vi "rqcBob QKey Processing.vi"(0 "rqcBob ServiceNET in":T1, 5 "Correct indices":u32[](array[numeric]), 7 "Raw Bob's data":u8[](array[numeric]), 9 "data valid":bool, 11 "error in":errorcluster) -> (4 "rqcBob ServiceNET out":T1, 6 "Incorrect Alice's data":bool, 8 "Bob's Key:":string="010100110101111110011011110000111111100101101001011100110010001011010011011001010000111101100001111011001111110010010110111100010001111011001000011001001101011000010111001010101110111010010000110011001101101100100101111100001111001011011110000010010101011001111010111001111100111110100100111011110001110101001100010011010001011011101010101000100011010101011010010001111110100010011010011001101101101000001100010110011001101001010101011000110010101100111101110101110011110100101100100001100100001101100001110010011000001101111001111110101101001010000110011100000011111101100010010100111000101011100110111010011100100000110000100110111101100000011011010011110000111011110111001101110001101011100111000010001001011000101100001110011001000100110101110010100000011011000001100111000101000100001110001001001011101100101101111000011101000111001110111000000101101000101011110101001101000001001000010011001010000011111111010010010001111011111001110001010100000010001000000101000000100101011010110100010111110111011110001100101010110010011101001010001100100000110000001111110101000001010000110001000011101110100110001000001100010101001000", 15 "error out":errorcluster)   [LabVIEW 2018]
uses:
  Shared/Shared Host Lib/rqc ServiceNET/Bob/Custom Controls/rqcBob ServiceNET control.ctl
  Shared/Shared Host Lib/rqc ServiceNET/Custom Controls/rqc ServiceNET command.ctl
  Shared/Shared Host Lib/rqc ServiceNET/Bob/rqcBob Send Data/rqcBob ServiceNET Send Data U8.vi
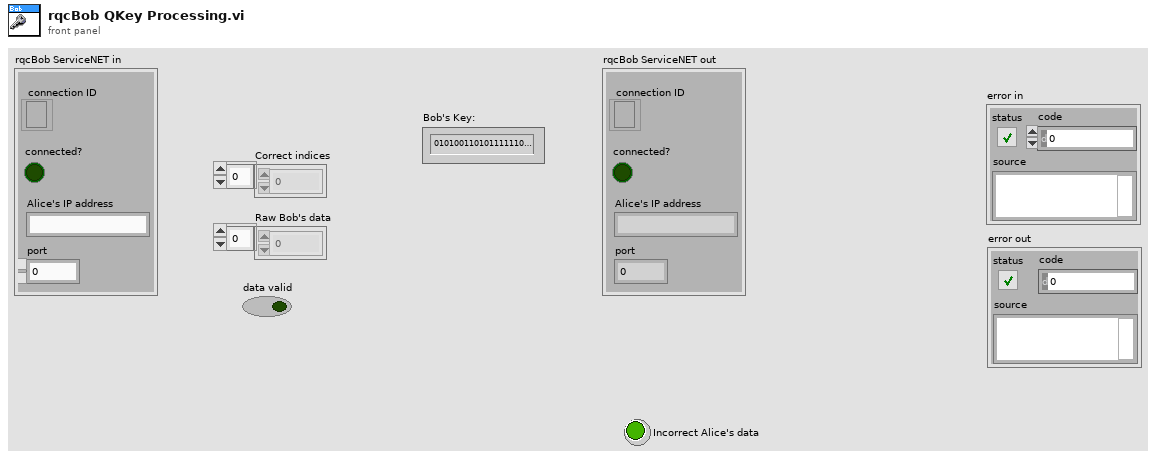
[diagram p1: front panel]
types:
  T1 = typedef "rqcBob ServiceNET control.ctl" = cluster{"connection ID":refnum<k5>, "connected?":bool, "Alice's IP address":string, "port":u16}
  T2 = typedef "rqc ServiceNET command.ctl" = enum8{"NONE", "READY", "START", "PING", "SEND KEY", "WRITE KEY", "WRITE AND SAVE KEY"}
  T3 = enum16{"open", "replace", "create", "open or create", "replace or create", "replace or create with confirmation"}
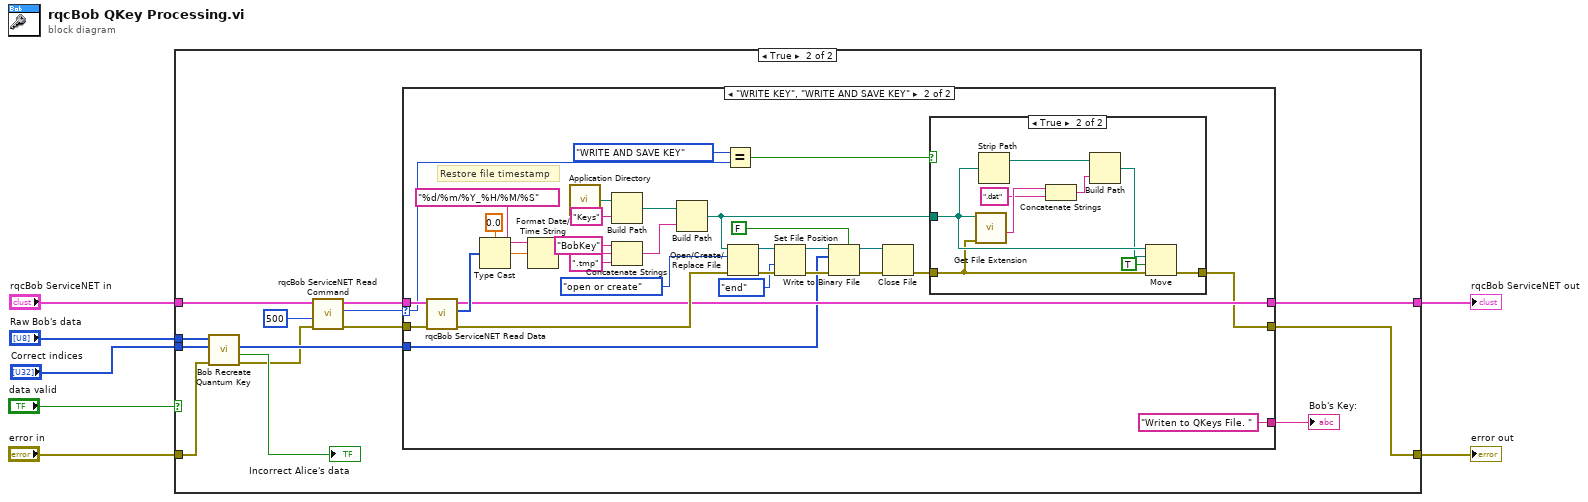
[diagram p0: block diagram]
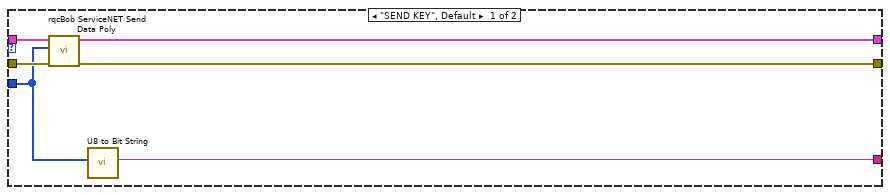
[diagram p3: hidden frame]
diagram:
  n1 = case shown="True" "data valid" {
    tunnel: "Raw Bob's data" -> [_ w23]
    tunnel: "Correct indices" -> [_ w22]
    tunnel: "error in" -> [w9 w21]
    tunnel: [w9 w18] -> w2
    tunnel: "rqcBob ServiceNET in" -> [w8 w16]
    tunnel: [w8 w19] -> w6
    frame False {
    }
    frame True {
      n2 = call "Bob Recreate Quantum Key.vi"("error in"=w21, "Correct Measurements Indexes in"=w22, "Raw Data in"=w23) -> ("error out"=w15:errorcluster, "Incorrect Alice's data"=→"Incorrect Alice's data":bool, "Sifted Key out"=w17:u8[])  [unwired: 6 in]
      n3 = call "rqcBob ServiceNET Read Command.vi"("error in"=w15, "timeout ms (50)"=500, "rqcBob ServiceNET in"=w16) -> ("error out"=w12:errorcluster, "command"=w14:T2, "rqcBob ServiceNET out"=w13:T1)  [unwired: 5 in, 1 out]
      n4 = case shown="\"WRITE KEY\", \"WRITE AND SAVE KEY\"" w14 {
        selector: w14 -> [_ w34]
        tunnel: [w29 w36] -> w19
        tunnel: [w28 w35] -> w18
        tunnel: w17 -> [w25 w31]
        tunnel: w13 -> [w27 w61]
        tunnel: w12 -> [w26 w60]
        tunnel: [w24 "Writen to QKeys File. " ("String out")] -> w11
        frame "SEND KEY", Default {
          n5 = call-poly "rqcBob ServiceNET Send Data Poly.vi"("error in"=w26, "Data"=w25, "rqcBob ServiceNET in"=w27) -> ("error out"=w28:errorcluster, "rqcBob ServiceNET out"=w29:T1)  [unwired: 7 in]
          n6 = call "U8 to Bit String.vi"("U8 in"=w25) -> ("String out"=w24:string)  [unwired: 10 in]
        }
        frame "WRITE KEY", "WRITE AND SAVE KEY" {
          # "Restore file timestamp"
          n7 = call "rqcBob ServiceNET Read Data.vi"("error in"=w60, "rqcBob ServiceNET in"=w61) -> ("error out"=w37:errorcluster, "Data"=w59:u32[], "rqcBob ServiceNET out"=w36:T1)  [unwired: 6 in, 1 out]
          n8 = Type Cast(type=0.0, x=w59) -> (*(type *) &x=w56:dbl)
          n9 = Format Date/Time String(time format string (%c)="%d/%m/%Y_%H/%M/%S", seconds (now)=w56) -> (date/time string=w55:string)  [unwired: 1 in]
          n10 = call <vilib>:"Application Directory.vi"() -> ("Application Directory"=w52:path)
          n11 = Build Path(base path=w52, name or relative path="Keys") -> (appended path=w49:path)
          n12 = Concatenate Strings("BobKey" ("string"), w55, ".tmp" ("string")) -> (w50:string)
          n13 = Build Path(base path=w49, name or relative path=w50) -> (appended path=w38:path)
          n14 = Equal?(x=rqc_ServiceNET_command."WRITE AND SAVE KEY", y=w34) -> (x = y?=w32:bool)
          n15 = Open/Create/Replace File(file path (use dialog)=w38, error in=w37, operation (0:open)=T3."open or create") -> (refnum out=w46:refnum<file>, error out=w44:errorcluster)  [unwired: 3 in, 1 out]
          n16 = Set File Position(refnum=w46, from (0:start)=enum16{"start", "end", "current"}."end", error in=w44) -> (refnum out=w45:refnum<file>, error out=w43:errorcluster)  [unwired: 1 in]
          n17 = Write to Binary File(file (use dialog)=w45, data=w31, error in=w43, 5:FALSE ("prepend array or string size? (T)")) -> (refnum out=w41:refnum<file>, error out=w40:errorcluster)  [unwired: 2 in, 1 out]
          n18 = Close File(refnum=w41, error in=w40) -> (error out=w39:errorcluster)  [unwired: 1 out]
          n19 = case shown="True" w32 {
            tunnel: w38 -> [_ w70]
            tunnel: w39 -> [w62 w69]
            tunnel: [w62 w63] -> w35
            frame False {
            }
            frame True {
              n20 = call <vilib>:"Get File Extension.vi"("error in (no error)"=w69, "file"=w70) -> ("filename without extension"=w68:string)  [unwired: 5 in, 4 out]
              n21 = Strip Path(path=w70) -> (stripped path=w71:path)  [unwired: 1 out]
              n22 = Concatenate Strings(w68, ".dat" ("string")) -> (w66:string)
              n23 = Build Path(base path=w71, name or relative path=w66) -> (appended path=w65:path)
              n24 = Move(source path=w70, error in=w69, 9:TRUE ("overwrite (F)"), 10:w65) -> (error out=w63:errorcluster)  [unwired: 1 in, 2 out]
            }
          }
        }
      }
      "Bob's Key:" <- w11
    }
  }
  "rqcBob ServiceNET out" <- w6
  "error out" <- w2
